vi "Sequence-StepComplete.vi"(0 "MCListbox Refnum":refnum<vi>, 5 "Step Feedback":T1, 11 "error in (no error)":errorcluster) -> (4 "MCListbox Refnum(dup)":refnum<vi>, 15 "error out":errorcluster)   [LabVIEW 2020, in "CSMStand(Lite).lvlib"]
uses:
  CSMStand(Lite).lvlib
  <vilib>/Utility/miscctls.llb/LVRowAndColumnTypeDef.ctl
  d146a9cb-ae7a-4dd4-bb46-4eefd7c37fd3.vi
  <userlib>/_NEVSTOP/Communicable State Machine(CSM)/addons/API-String-Arugments-Support/_Support/Data To API String Arguments.vi
  <userlib>/NEVSTOP-Programming-Palette/Dialog & Interface/_support/Autosize All MultiListbox Columns (Uniform Text)_nevstop.vi
panel:
  # "Connector Pane"
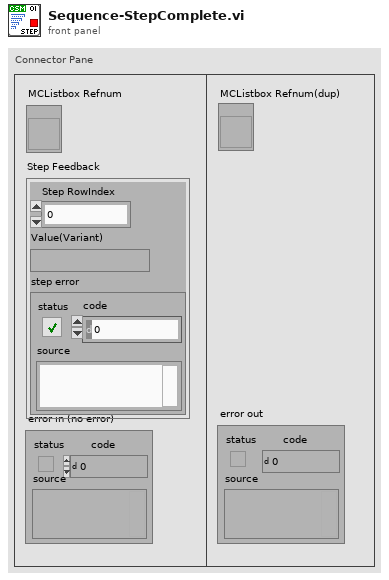
[diagram p1: front panel]
types:
  T1 = cluster{"Step RowIndex":i32, "Value(Variant)":variant, "step error":errorcluster}
  T2 = typedef "LVRowAndColumnTypeDef.ctl" = cluster{"Row":i32, "Column":i32}
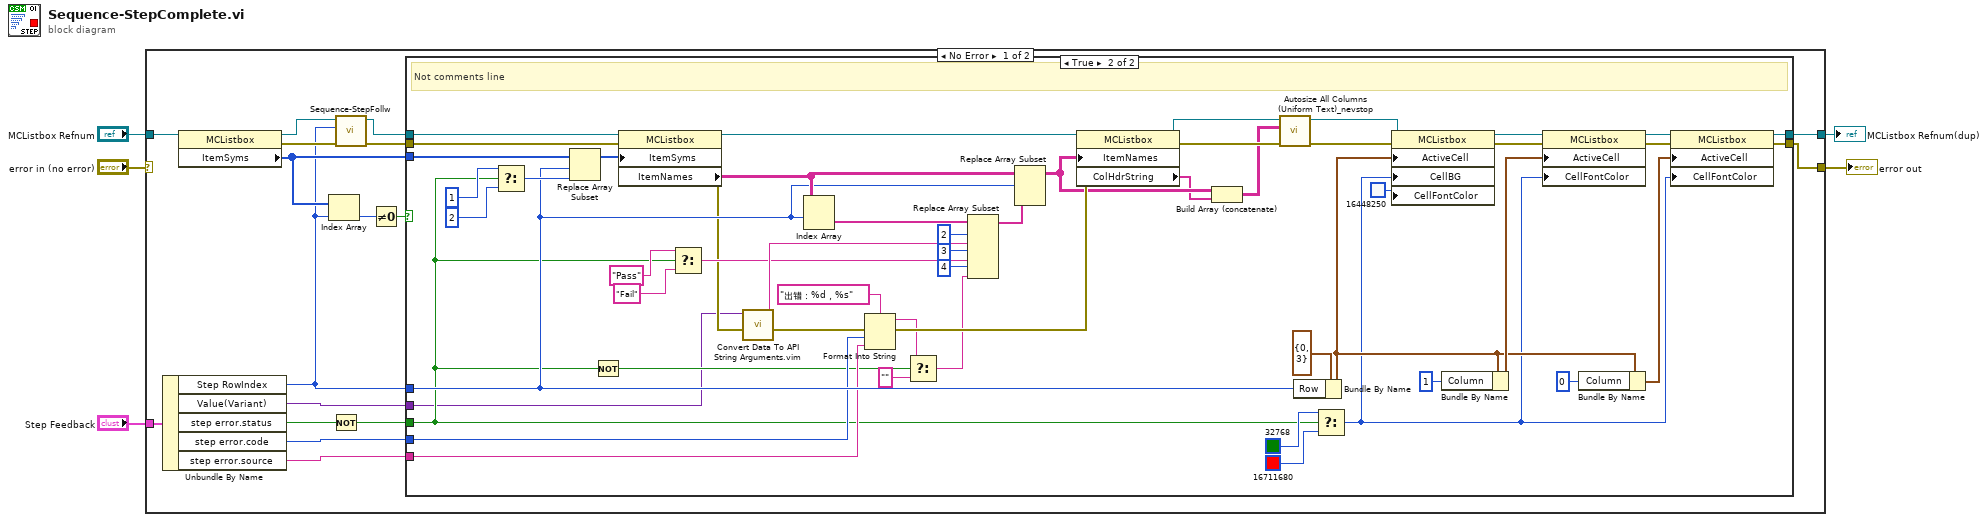
[diagram p0: block diagram]
diagram:
  n1 = case shown="No Error" "error in (no error)" {
    selector: "error in (no error)" -> [_ w80]
    tunnel: [w20 w80] -> w5
    tunnel: "MCListbox Refnum" -> [w22 w79]
    tunnel: [w21 w79] -> w2
    tunnel: "Step Feedback" -> [w14 _]
    frame No Error {
      n2 = Unbundle By Name(w14) -> ("Step RowIndex"=w6:i32, "Value(Variant)"=w16:variant, "step error.status"=w15:bool, "step error.code"=w13:i32, "step error.source"=w12:string)
      n3 = property class="MCListbox"(reference=w22) -> (reference out=w8:refnum<vi>, error out=w10:errorcluster, "ItemSyms"=w19:i32[])  [unwired: 1 in]
      n4 = Index Array(array=w19, index=w6) -> (element=w18:i32)
      n5 = Not(x=w15) -> (.not. x?=w11:bool)
      n6 = call "Sequence-StepFollw.vi"("error in (no error)"=w10, "Row Index"=w6, "MCListbox Refnum"=w8) -> ("error out"=w9:errorcluster, "MCListbox Refnum(dup)"=w7:refnum<vi>)  [unwired: 7 in]
      n7 = Not Equal To 0?(x=w18) -> (x != 0?=w17:bool)
      n8 = case shown="True" w17 {
        tunnel: [w24 w33] -> w21
        tunnel: [w23 w30] -> w20
        tunnel: w7 -> [w24 w77]
        tunnel: w9 -> [w23 w72]
        tunnel: w11 -> [_ w45]
        tunnel: w19 -> [_ w68]
        tunnel: w6 -> [_ w59]
        tunnel: w16 -> [_ w25]
        tunnel: w13 -> [_ w48]
        tunnel: w12 -> [_ w47]
        frame False {
        }
        frame True {
          # "Not comments line"
          n9 = Select(t=1 ("Step RowIndex"), s=w45, f=2 ("Step RowIndex")) -> (s? t:f=w74:i32)
          n10 = Replace Array Subset(array=w68, new element=w74, index=w59) -> (w71:i32[])
          n11 = Not(x=w45) -> (.not. x?=w41:bool)
          n12 = property class="MCListbox"(reference=w77, error in=w72, "ItemSyms"=w71) -> (reference out=w73:refnum<vi>, error out=w56:errorcluster, "ItemNames"=w60:string[][])
          n13 = Select(t="Pass", s=w45, f="Fail") -> (s? t:f=w63:string)
          n14 = call "Convert Data To API String Arguments.vim"("error in (no error)"=w56, "data"=w25) -> ("error out"=w50:errorcluster, "String"=w64:string)  [unwired: 6 in]
          n15 = Index Array(array=w60, index (row)=w59) -> (element=w67:string[])  [unwired: 1 in]
          n16 = Format Into String(format string="出错：%d，%s", error in=w50, w48, w47) -> (resulting string=w44:string, error out=w49:errorcluster)  [unwired: 1 in]
          n17 = Select(t=w44, s=w41, f="") -> (s? t:f=w42:string)
          n18 = Replace Array Subset(array=w67, new element #1=w64, index #1=2 ("index"), new element #2=w63, index #2=3 ("index"), new element #3=w42, index #3=4 ("index")) -> (w58:string[])
          n19 = Replace Array Subset(array=w60, new element=w58, index (row)=w59) -> (w40:string[][])  [unwired: 1 in]
          n20 = property class="MCListbox"(reference=w73, error in=w49, "ItemNames"=w40) -> (reference out=w53:refnum<vi>, error out=w55:errorcluster, "ColHdrString"=w39:string[])
          n21 = Build Array (concatenate)(w40, w39) -> (w38:string[][])
          n22 = call-poly <userlib>:"Autosize All Columns (Uniform Text)_nevstop.vi"("error in (no error)"=w55, "Array"=w38, "Control in"=w53) -> ("error out"=w54:errorcluster, "Control in"=w52:refnum<vi>)  [unwired: 7 in]
          n23 = Bundle By Name(cluster=T2 {"Row"=0, "Column"=3} ("Active Cell:Active Cell"), "Row"=w59) -> (w29:T2)
          n24 = Select(t=u32 32768 ("Active Cell:Cell Font:Color"), s=w45, f=u32 16711680 ("Active Cell:Cell Font:Color")) -> (s? t:f=w27:u32)
          n25 = property class="MCListbox"(reference=w52, error in=w54, "ActiveCell"=w29, "CellBG"=w27, "CellFontColor"=u32 16448250 ("Active Cell:Cell Font:Color")) -> (reference out=w37:refnum<vi>, error out=w36:errorcluster)
          n26 = Bundle By Name(cluster=w29, "Column"=1) -> (w34:T2)
          n27 = property class="MCListbox"(reference=w37, error in=w36, "ActiveCell"=w34, "CellFontColor"=w27) -> (reference out=w32:refnum<vi>, error out=w31:errorcluster)
          n28 = Bundle By Name(cluster=w29, "Column"=0) -> (w26:T2)
          n29 = property class="MCListbox"(reference=w32, error in=w31, "ActiveCell"=w26, "CellFontColor"=w27) -> (reference out=w33:refnum<vi>, error out=w30:errorcluster)
        }
      }
    }
    frame Error {
    }
  }
  "error out" <- w5
  "MCListbox Refnum(dup)" <- w2
